vi "Configure Dialog.vi"(8 "error in (no error)":errorcluster, 11 "Configure Arbitrary Waveform [ARB] Msg in":refnum<class "Configure Arbitrary Waveform [ARB] Msg.lvclass">) -> (0 "error out":errorcluster, 2 "Ok?":bool, 3 "Configure Arbitrary Waveform [ARB] Msg out":refnum<class "Configure Arbitrary Waveform [ARB] Msg.lvclass">)   [LabVIEW 2014, in "CS++Fgen.lvlib" / "Configure Arbitrary Waveform [ARB] Msg.lvclass"]
uses:
  Configure Arbitrary Waveform [ARB] Msg.lvclass
  CSPP_Core/Actors/CS++PVMonitor Messages/CS++PVUpdate Msg/CS++PVUpdate Msg.lvclass
panel:
  in  "waveform handle (0)":i32 caption="Waveform Handle"
  in  "gain (1.00)":dbl=1.0 caption="Gain" format="%.4f"
  in  "offset (0.00 V)":dbl[unit] caption="Offset" format="%.4f"
  in  "channel name (\"CHANNEL1\")":string="CHANNEL1" caption="Channel Name"
  in  "OK Button":bool
  in  "Cancel Button":bool
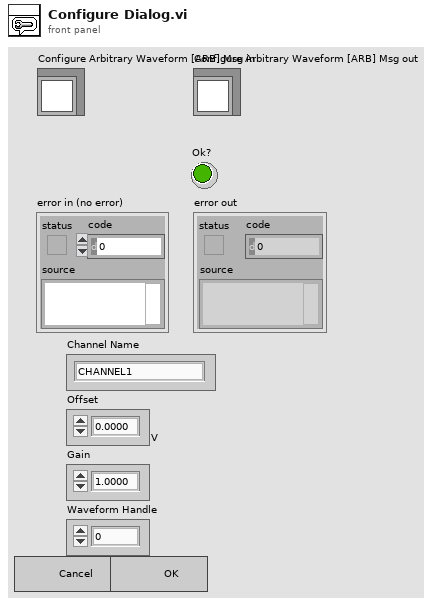
[diagram p1: front panel]
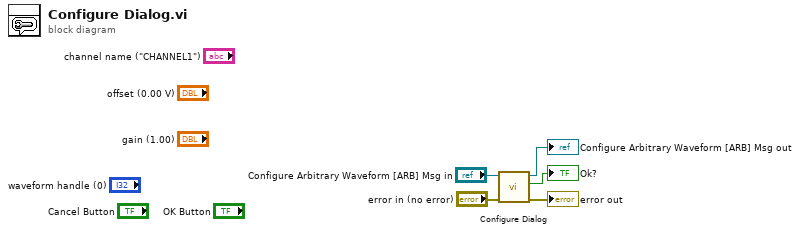
[diagram p0: block diagram]
diagram:
  n1 = call-parent "Configure Dialog.vi"("error in (no error)"="error in (no error)", "Message in"="Configure Arbitrary Waveform [ARB] Msg in") -> ("error out"=→"error out":errorcluster, "Ok?"=→"Ok?":bool, "Message out"=→"Configure Arbitrary Waveform [ARB] Msg out":refnum<class "Configure Arbitrary Waveform [ARB] Msg.lvclass">)  [unwired: 7 in]
